vi "Save Action.vi"(8 "error in (no error)":errorcluster, 9 "Signal":dbl[](graph), 10 "Saving Parameters":T1, 11 "Function Generator Actor in":refnum<class "Function Generator Actor.lvclass">) -> (0 "error out":errorcluster, 3 "Function Generator Actor out":refnum<class "Function Generator Actor.lvclass">)   [LabVIEW 2020, in "Function Generator Actor.lvlib" / "Function Generator Actor.lvclass"]
uses:
  Function Generator Actor.lvclass
  C:/Program Files (x86)/National Instruments/LabVIEW 2020/vi.lib/ActorFramework/Actor/Actor.lvclass
  CSV Logging/CSV Logging/CSV Logging.lvclass
  Plain Text Logging/Plain Text Logging/Plain Text Logging.lvclass
  TDMS Logging/TDMS Logging/TDMS Logging.lvclass
  <vilib>/ActorFramework/Actor/Actor.lvclass/Actor.ctl
  <vilib>/ActorFramework/Message Enqueuer/Message Enqueuer.lvclass/Message Enqueuer.ctl
  Function Generator Actor.lvclass/Function Generator Actor.ctl
  Function Generator Actor Messages/Get File Name Msg/Get File Name Msg.lvclass/Get File Name Msg.ctl
  Saving Actor/Saving Actor Messages/SaveData Msg/SaveData Msg.lvclass/SaveData Msg.ctl
  <vilib>/ActorFramework/Message Enqueuer/Init from Existing Queue.vi
  <vilib>/ActorFramework/Message Enqueuer/Enqueue.vi
  Saving Actor/Saving Actor/Saving Actor.lvclass
  Function Generator Actor Messages/Get File Name Msg/Get File Name Msg.lvclass
  C:/Program Files (x86)/National Instruments/LabVIEW 2020/vi.lib/ActorFramework/Message/Message.lvclass
  Saving Actor/Saving Actor Messages/SaveData Msg/SaveData Msg.lvclass
  <vilib>/ActorFramework/Message Priority Queue/Priority Enqueue.vi
  <vilib>/ActorFramework/Message Enqueuer/Message Enqueuer.lvclass
  <vilib>/ActorFramework/Actor/Actor.lvclass
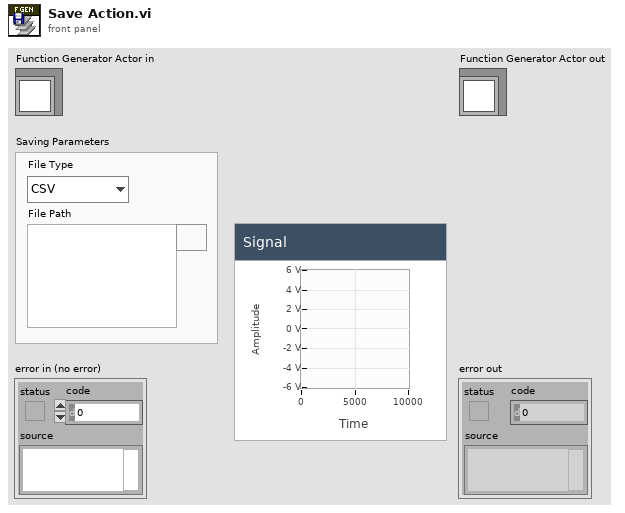
[diagram p1: front panel]
types:
  T1 = cluster{"File Type":enum16{"CSV", "Plain Text", "TDMS"}, "File Path":path}
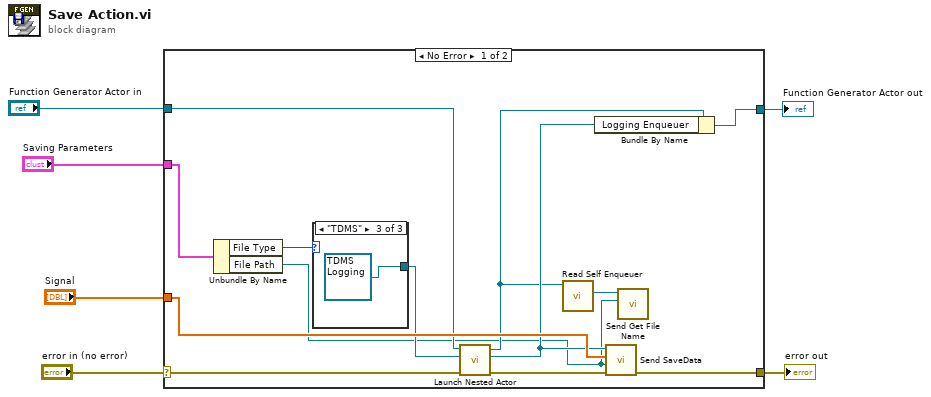
[diagram p0: block diagram]
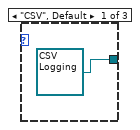
[diagram p2: hidden frame]
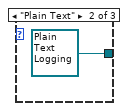
[diagram p3: hidden frame]
diagram:
  n1 = case shown="No Error" "error in (no error)" {
    selector: "error in (no error)" -> [w19 w24]
    tunnel: [w15 w24] -> w5
    tunnel: "Saving Parameters" -> [w18 _]
    tunnel: "Signal" -> [w14 _]
    tunnel: "Function Generator Actor in" -> [w11 w23]
    tunnel: [w10 w23] -> w1
    frame No Error {
      n2 = Unbundle By Name(w18) -> ("File Type"=w17:enum16{"CSV", "Plain Text", "TDMS"}, "File Path"=w7:path)
      n3 = case shown="\"TDMS\"" w17 {
        tunnel: [refnum<class "CSV Logging.lvclass"> refnum ("CSV Logging.lvlib:CSV Logging.lvclass") refnum<class "Plain Text Logging.lvclass"> refnum ("Plain Text Logging.lvlib:Plain Text Logging.lvclass") refnum<class "TDMS Logging.lvclass"> refnum ("TDMS Logging.lvlib:TDMS Logging.lvclass")] -> w13
        frame "CSV", Default {
        }
        frame "Plain Text" {
        }
        frame "TDMS" {
        }
      }
      n4 = call <vilib>:"Launch Nested Actor.vi"("error in (no error)"=w19, "Nested Actor"=w13, "Caller Actor in"=w11) -> ("error out"=w16:errorcluster, "Nested Actor's Enqueuer"=w12:refnum<class "Message Enqueuer.lvclass">, "Caller Actor out"=w8:refnum<class "Function Generator Actor.lvclass">)  [unwired: 6 in]
      n5 = call <vilib>:"Read Self Enqueuer.vi"("Actor"=w8) -> ("Self Enqueuer"=w9:refnum<class "Message Enqueuer.lvclass">)  [unwired: 10 in]
      n6 = Bundle By Name(cluster=w8, "Logging Enqueuer"=w12) -> (w10:refnum<class "Function Generator Actor.lvclass">)
      n7 = call "Send SaveData.vi"("error in (no error)"=w16, "Path Control"=w7, "Signal"=w14, "Message Enqueuer"=w12) -> ("error out"=w15:errorcluster)  [unwired: 6 in, 1 out]
      n8 = call "Send Get File Name.vi"("Path"=w7, "Message Enqueuer"=w9) -> ()  [unwired: 8 in, 2 out]
    }
    frame Error {
    }
  }
  "error out" <- w5
  "Function Generator Actor out" <- w1
